vi "Do.vi"(8 "error in (no error)":errorcluster, 10 "Actor in":refnum<class "Actor.lvclass">, 11 "Integrate Pulse Msg":refnum<class "Integrate Pulse Msg.lvclass">) -> (0 "error out":errorcluster, 2 "Actor out":refnum<class "Actor.lvclass">)   [LabVIEW 2019, in "DigitiserActor.lvlib" / "Integrate Pulse Msg.lvclass"]
doc: "This VI delivers the message to the actor by calling the appropriate method(s) on the actor."
uses:
  Integrate Pulse Msg.lvclass
  <vilib>/ActorFramework/Actor/Actor.lvclass
  DigitiserActor/DigitiserActor.lvclass
  C:/Program Files (x86)/National Instruments/LabVIEW 2019/vi.lib/ActorFramework/Actor/Actor.lvclass
  Integrate Pulse Msg.lvclass/Integrate Pulse Msg.ctl
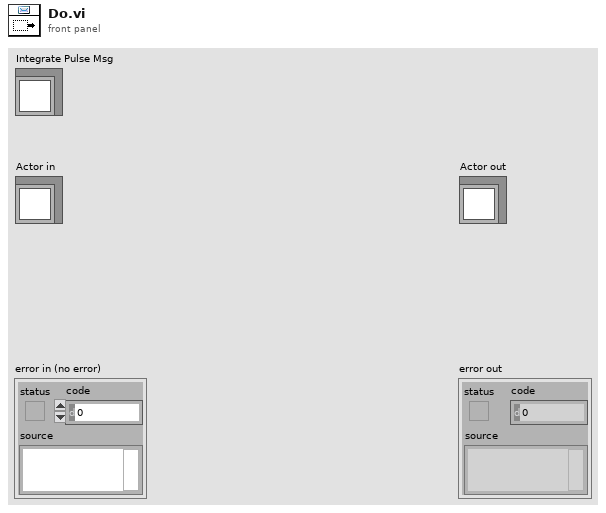
[diagram p1: front panel]
types:
  T1 = cluster{"PSD refnum":refnum<vi>, "Q_short refnum":refnum<vi>, "Q_long refnum":refnum<vi>}
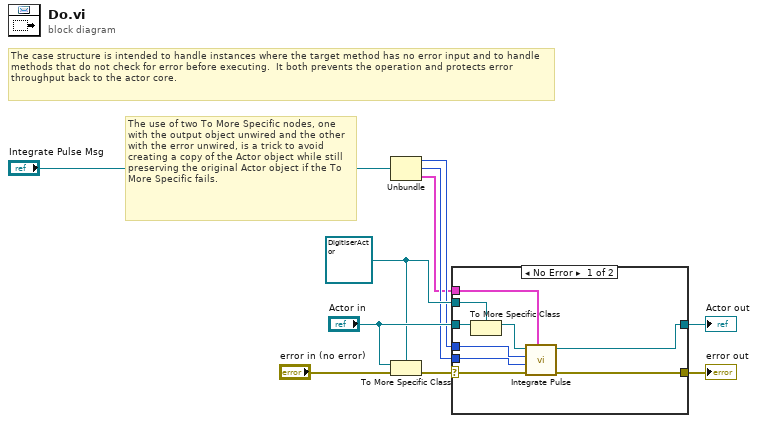
[diagram p0: block diagram]
diagram:
  w5 = refnum<class "DigitiserActor.lvclass"> refnum ("Actor in")
  # "The use of two To More Specific nodes, one with the output object unwired and the other with the error unwired, is a trick to avoid creating a copy of the Actor object while still preserving the original Actor object if the To More Specific fails."
  # "The case structure is intended to handle instances where the target method has no error input and to handle methods that do not check for error before executing.  It both prevents the operation and protects error throughput back to the actor core."
  n1 = Unbundle("Integrate Pulse Msg") -> (w3:i32, w2:i32, w1:T1)
  n2 = To More Specific Class(target class=w5, reference="Actor in", error in="error in (no error)") -> (error out=w4:errorcluster)  [unwired: 1 out]
  n3 = case shown="No Error" w4 {
    selector: w4 -> [w17 w21]
    tunnel: [w19 w21] -> w10
    tunnel: [w18 w20] -> w9
    tunnel: "Actor in" -> [w16 w20]
    tunnel: w5 -> [w15 _]
    tunnel: w3 -> [w13 _]
    tunnel: w2 -> [w12 _]
    tunnel: w1 -> [w11 _]
    frame No Error {
      n4 = To More Specific Class(target class=w15, reference=w16) -> (specific class reference=w14:refnum<class "DigitiserActor.lvclass">)  [unwired: 1 in, 1 out]
      n5 = call-dynamic "Integrate Pulse.vi"("Refnum Cluster in"=w11, "error in (no error)"=w17, "Short Gate in"=w12, "Long Gate in"=w13, "DigitiserActor in"=w14) -> ("error out"=w19:errorcluster, "DigitiserActor out"=w18:refnum<class "DigitiserActor.lvclass">)  [unwired: 5 in]
    }
    frame Error {
      # "If type check fails, pass the original object out again."
    }
  }
  "error out" <- w10
  "Actor out" <- w9
